vi "test-slew-rate-limiter-2.vi"() -> ()   [LabVIEW 2019]
uses:
  <vilib>/Rock Robotics/WPI/ThirdParty/JAS_Junk/TrajLib/Trajectory_Library.lvlib
panel:
  out "T1 = 0.5":dbl
  out "T0 -- < 2":dbl
  # "Slew Rate Limiter Test"
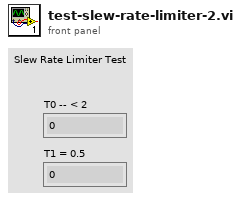
[diagram p1: front panel]
types:
  T1 = typedef "Trajectory_Library.lvlib/SLEW_RATE_LIMITER.ctl" = cluster{"RateLimit":dbl, "PrevValue":dbl, "Timer":T2}
  T2 = typedef "Trajectory_Library.lvlib/TIMER.ctl" = cluster{"StartTime":dbl, "Accumulated TIme":dbl, "Running":bool, "semaphore":T3}
  T3 = typedef "Semaphore RefNum" = refnum<k1>
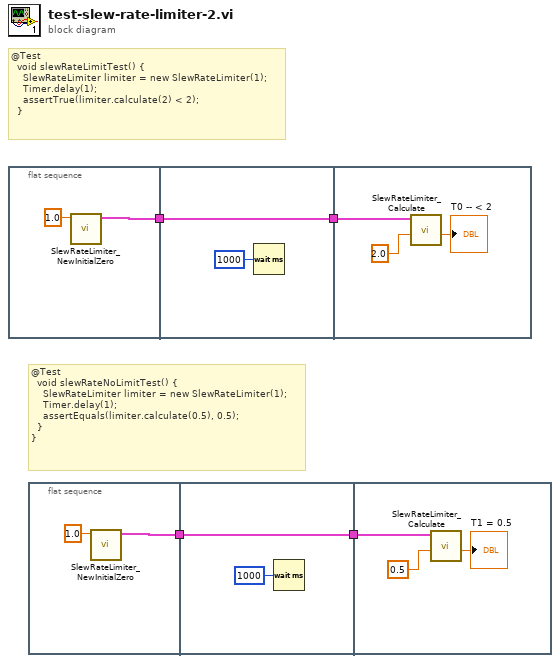
[diagram p0: block diagram]
diagram:
  # "@Test\n  void slewRateNoLimitTest() {\n    SlewRateLimiter limiter = new SlewRateLimiter(1);\n    Timer.delay(1);\n    assertEquals(limiter.calculate(0.5), 0.5);\n  }\n}"
  # "@Test\n  void slewRateLimitTest() {\n    SlewRateLimiter limiter = new SlewRateLimiter(1);\n    Timer.delay(1);\n    assertTrue(limiter.calculate(2) < 2);\n  }"
  n1 = flat-sequence {
    tunnel: [w5] -> w4
    tunnel: w4 -> [w7]
    tunnel: [w7] -> w3
    tunnel: w3 -> [w10]
    frame #0 {
      n2 = call <vilib>:"SlewRateLimiter_NewInitialZero.vi"("RateLimit"=1.0) -> ("out SLEW_RATE_LIMITER"=w5:T1)  [unwired: 10 in]
    }
    frame #1 {
      n3 = Wait (ms)(milliseconds to wait=u32 1000) -> ()  [unwired: 1 out]
    }
    frame #2 {
      n4 = call <vilib>:"SlewRateLimiter_Calculate.vi"("Input"=2.0, "in SLEW_RATE_LIMITER"=w10) -> ("Output"=→"T0 -- < 2":dbl)  [unwired: 8 in, 1 out]
    }
  }
  n5 = flat-sequence {
    tunnel: [w12] -> w2
    tunnel: w2 -> [w14]
    tunnel: [w14] -> w1
    tunnel: w1 -> [w17]
    frame #0 {
      n6 = call <vilib>:"SlewRateLimiter_NewInitialZero.vi"("RateLimit"=1.0) -> ("out SLEW_RATE_LIMITER"=w12:T1)  [unwired: 10 in]
    }
    frame #1 {
      n7 = Wait (ms)(milliseconds to wait=u32 1000) -> ()  [unwired: 1 out]
    }
    frame #2 {
      n8 = call <vilib>:"SlewRateLimiter_Calculate.vi"("Input"=0.5, "in SLEW_RATE_LIMITER"=w17) -> ("Output"=→"T1 = 0.5":dbl)  [unwired: 8 in, 1 out]
    }
  }
